vi "Periodic Tasks.vi"() -> ()   [LabVIEW 2017]
doc: "This VI runs in parallel to other tasks. It can contain as many user-defined periodic loops as you need. These can carry out PID or other sorts of timed response."
uses:
  TankDrivePreseason/RightMotors.ctl
  TankDrivePreseason/LeftMotors.ctl
  <vilib>/Rock Robotics/WPI/ThirdParty/Phoenix-LabVIEW/Motor Controller/Controls/CTRE_Phoenix_MotorControl_ControlMode.ctl
  <vilib>/Rock Robotics/WPI/ThirdParty/Phoenix-LabVIEW/Pigeon IMU/CTRE_PigeonIMU_GetYPR.vi
  <vilib>/addons/control/pid/pid.llb/PID (DBL).vi
  Robot Global Data.vi
  <vilib>/addons/control/pid/NI_PID_pid.lvlib
panel:
  in  "motor cap":dbl
  in  "PID output range":cluster{"output high":dbl, "output low":dbl}={"output high"=100.0, "output low"=-100.0} {"output low" format="%.2f"; "output high" format="%.2f"}
  in  "Pigeon PID gains":T1={"proportional gain (Kc)"=1.0, "integral time (Ti, min)"=0.01, "derivative time (Td, min)"=0.0} {"derivative time (Td, min)" format="%.3f"; "integral time (Ti, min)" format="%.3f"; "proportional gain (Kc)" format="%.3f"}
  in  "error in":errorcluster
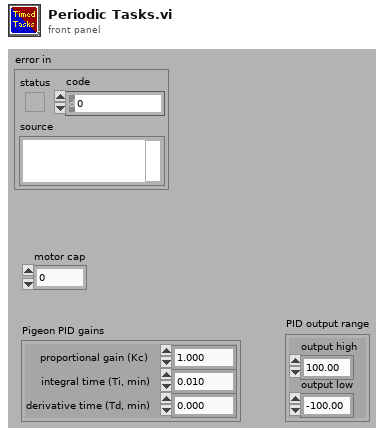
[diagram p1: front panel]
types:
  T1 = cluster{"proportional gain (Kc)":dbl, "integral time (Ti, min)":dbl, "derivative time (Td, min)":dbl}
  T2 = typedef "LeftMotors.ctl" = enum16{"LMotor 1", "LMotor 2", "LMotor 3"}
  T3 = typedef "RightMotors.ctl" = enum16{"RMotor 1", "RMotor 2", "RMotor 3"}
  T4 = typedef "WPI_MotorControlDeviceRef.ctl" = cluster{"DeviceStatus":errorcluster, "Type":T5, "PWM":cluster{"PWM Channel":T6, "DeadBand":T7}, "CAN":cluster{"Device Number":u8, "SetOutput VI Ref":variant, "GetOutput VI Ref":variant, "Enable VI Ref":variant, "Disable VI Ref":variant, "Data":variant}, "Invert":bool, "DIO PWM":cluster{"PWM \"Enable\" Channel":T6, "DIOChannel":T8, "PWM Rate":dbl}}
  T5 = typedef "WPI_MotorControlType.ctl" = enum16{"PWM", "CAN", "DIO PWM"}
  T6 = typedef "FPGA_DIOPWMChannel.ctl" = enum8{"PWM 0", "PWM 1", "PWM 2", "PWM 3", "PWM 4", "PWM 5", "PWM 6", "PWM 7", "PWM 8", "PWM 9", "PWM MXP 0", "PWM MXP 1", "PWM MXP 2", "PWM MXP 3", "PWM MXP 4", "PWM MXP 5", "PWM MXP 6", "PWM MXP 7", "PWM MXP 8", "PWM MXP 9", "Invalid"}
  T7 = typedef "WPI_PWMDeadband.ctl" = cluster{"Name":string, "maxPositivePwm":i32, "minPositivePwm":i32, "centerPwm":i32, "maxNegativePwm":i32, "minNegativePwm":i32, "angularRange":u16}
  T8 = typedef "FPGA_DIOChannel.ctl" = enum8{"DIO 0", "DIO 1", "DIO 2", "DIO 3", "DIO 4", "DIO 5", "DIO 6", "DIO 7", "DIO 8", "DIO 9", "DIO MXP 0", "DIO MXP 1", "DIO MXP 2", "DIO MXP 3", "DIO MXP 4", "DIO MXP 5", "DIO MXP 6", "DIO MXP 7", "DIO MXP 8", "DIO MXP 9", "DIO MXP 10", "DIO MXP 11", "DIO MXP 12", "DIO MXP 13", "DIO MXP 14", "DIO MXP 15", "SPI Port CS1", "SPI Port CS2", "SPI Port CS3", "SPI Port MISO", "SPI Port MOSI", "Invalid"}
  T9 = typedef "CTRE_PigeonIMU_DeviceRef.ctl" = cluster{"DeviceStatus":errorcluster, "Device Number":u8, "Type":T10, "Device ID":u32, "Handle":u64, "UsageFrame":u32, "Library Path":path}
  T10 = typedef "CTRE_PigeonIMU_ConnectionType.ctl" = u32
  T11 = typedef "CTRE_Phoenix_MotorControl_ControlMode.ctl" = u16
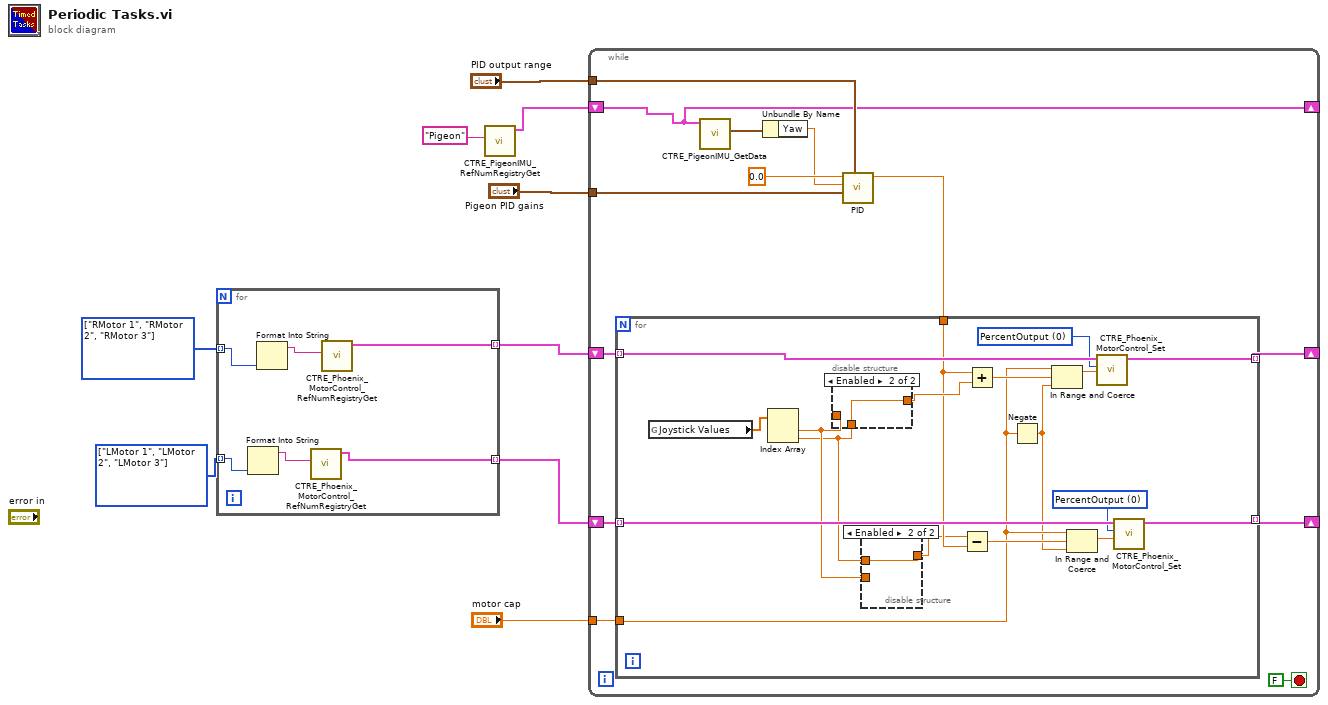
[diagram p0: block diagram]
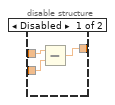
[diagram p2: hidden frame]
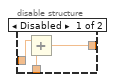
[diagram p3: hidden frame]
diagram:
  w8 = T2[] [enum."LMotor 1", enum."LMotor 2", enum."LMotor 3"] items=["LMotor 1", "LMotor 2", "LMotor 3"]
  w9 = T3[] [enum."RMotor 1", enum."RMotor 2", enum."RMotor 3"] items=["RMotor 1", "RMotor 2", "RMotor 3"]
  n1 = for {
    tunnel: w9 -> [w15] mode=indexing
    tunnel: w8 -> [w13] mode=indexing
    tunnel: [w11] -> w6 mode=indexing
    tunnel: [w10] -> w7 mode=indexing
    n2 = Format Into String(w13) -> (resulting string=w12:string)  [unwired: 3 in, 1 out]
    n3 = Format Into String(w15) -> (resulting string=w14:string)  [unwired: 3 in, 1 out]
    n4 = call <vilib>:"CTRE_Phoenix_MotorControl_RefNumRegistryGet.vi"("refnum name"=w12) -> ("PhoenixMotorControlDevRef"=w11:T4)  [unwired: 9 in, 1 out]
    n5 = call <vilib>:"CTRE_Phoenix_MotorControl_RefNumRegistryGet.vi"("refnum name"=w14) -> ("PhoenixMotorControlDevRef"=w10:T4)  [unwired: 9 in, 1 out]
  }
  n6 = call "CTRE_PigeonIMU_RefNumRegistryGet.vi"("refnum name"="Pigeon") -> ("PigeonIMUDevRef"=w2:T9)  [unwired: 9 in, 1 out]
  n7 = while {
    shift-right: [w26] -> _
    shift-left: w7 -> [w28]
    shift-right: [w25] -> _
    shift-left: w6 -> [w27]
    tunnel: "PID output range" -> [w23]
    tunnel: "Pigeon PID gains" -> [w22]
    tunnel: "motor cap" -> [w17]
    shift-right: [w16] -> _
    shift-left: w2 -> [w16]
    stop <- FALSE stop-if-true
    n8 = call-poly <vilib>:"CTRE_PigeonIMU_GetData.vi"("PigeonIMUDevRef"=w16) -> ("Yaw Pitch Roll"=w20:cluster{"Yaw":dbl, "Pitch":dbl, "Roll":dbl})  [unwired: 8 in, 2 out]
    n9 = Unbundle By Name(w20) -> ("Yaw"=w19:dbl)
    n10 = call-poly <vilib>:"PID.vi"("output range"=w23, "PID gains"=w22, "process variable"=w19, "setpoint"=0.0) -> ("output"=w18:dbl)  [unwired: 6 in, 1 out]
    n11 = for {
      tunnel: w28 -> [w46] mode=indexing
      tunnel: w27 -> [w45] mode=indexing
      tunnel: [w42] -> w26 mode=indexing
      tunnel: [w41] -> w25 mode=indexing
      tunnel: w18 -> [w31]
      tunnel: w17 -> [w33]
      w39 = T11 0 items=["PercentOutput"=0, "Position"=1, "Velocity"=2, "Current"=3, "Follower"=5, "MotionProfile"=6, "MotionMagic"=7, "MotionMagicArc"=8, "MotionProfileArc"=10, "Disabled"=15] ("Control Mode")
      w40 = T11 0 items=["PercentOutput"=0, "Position"=1, "Velocity"=2, "Current"=3, "Follower"=5, "MotionProfile"=6, "MotionMagic"=7, "MotionMagicArc"=8, "MotionProfileArc"=10, "Disabled"=15] ("Control Mode")
      n12 = global read "Robot Global Data.vi" "Joystick Values"() -> (w29:dbl[])
      n13 = Index Array(array=w29) -> (element #1=w44:dbl, element #2=w43:dbl)  [unwired: 2 in]
      n14 = disable-structure shown="Enabled" {
        disable-tunnel: w44 -> [w53 _]
        disable-tunnel: w43 -> [w52 w54]
        disable-tunnel: [w51 w54] -> w38
        frame Disabled {
          n15 = Add(x=w53, y=w52) -> (x+y=w51:dbl)
        }
        frame Enabled {
        }
      }
      n16 = disable-structure shown="Enabled" {
        disable-tunnel: w44 -> [w49 _]
        disable-tunnel: w43 -> [w48 w50]
        disable-tunnel: [w47 w50] -> w30
        frame Disabled {
          n17 = Subtract(x=w48, y=w49) -> (x-y=w47:dbl)
        }
        frame Enabled {
        }
      }
      n18 = Subtract(x=w30, y=w31) -> (x-y=w35:dbl)
      n19 = Add(x=w31, y=w38) -> (x+y=w37:dbl)
      n20 = Negate(x=w33) -> (-x=w32:dbl)
      n21 = In Range and Coerce(upper limit=w33, x=w37, lower limit=w32) -> (coerced(x)=w36:dbl)  [unwired: 1 out]
      n22 = In Range and Coerce(upper limit=w33, x=w35, lower limit=w32) -> (coerced(x)=w34:dbl)  [unwired: 1 out]
      n23 = call <vilib>:"CTRE_Phoenix_MotorControl_Set.vi"("Output"=w36, "Control Mode"=w40, "PhoenixMotorControlDevRef"=w46) -> ("PhoenixMotorControlDevRef"=w42:T4)  [unwired: 7 in, 1 out]
      n24 = call <vilib>:"CTRE_Phoenix_MotorControl_Set.vi"("Output"=w34, "Control Mode"=w39, "PhoenixMotorControlDevRef"=w45) -> ("PhoenixMotorControlDevRef"=w41:T4)  [unwired: 7 in, 1 out]
    }
  }
